vi "StartDataCollection.vi"   [LabVIEW 2011]
uses:
  GlobalVariables.vi
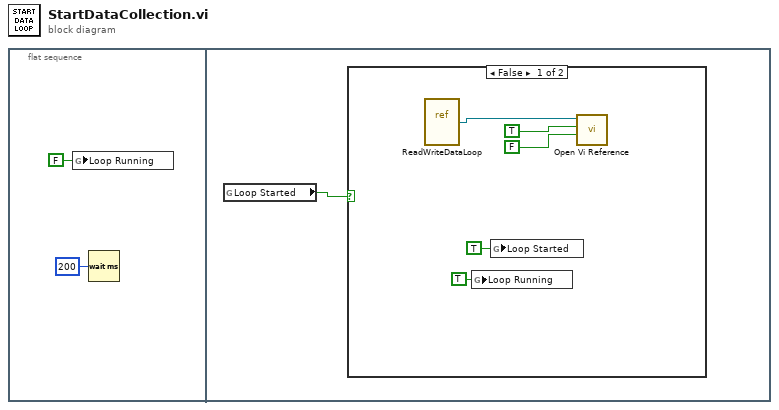
[diagram p0: block diagram]
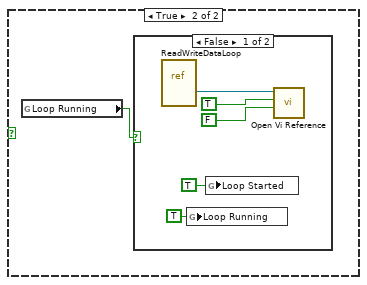
[diagram p2: hidden frame]
diagram:
  n1 = flat-sequence {
    frame #0 {
      n2 = global write "GlobalVariables.vi" "Loop Running"(FALSE ("Loop Running")) -> ()
      n3 = Wait (ms)(milliseconds to wait=u32 200) -> ()  [unwired: 1 out]
    }
    frame #1 {
      n4 = global read "GlobalVariables.vi" "Loop Started"() -> (w3:bool)
      n5 = case shown="False" w3 {
        frame False {
          n6 = vi-ref "ReadWriteDataLoop.vi"() -> (w6:refnum<vi>)
          n7 = global write "GlobalVariables.vi" "Loop Running"(TRUE ("Loop Started")) -> ()
          n8 = global write "GlobalVariables.vi" "Loop Started"(TRUE ("Loop Started")) -> ()
          n9 = call "Open Vi Reference.vi"("Show"=FALSE, "RunVi"=TRUE, "reference"=w6) -> ()  [unwired: 1 in, 2 out]
        }
        frame True {
          n10 = global read "GlobalVariables.vi" "Loop Running"() -> (w9:bool)
          n11 = case shown="False" w9 {
            frame False {
              n12 = vi-ref "ReadWriteDataLoop.vi"() -> (w12:refnum<vi>)
              n13 = global write "GlobalVariables.vi" "Loop Running"(TRUE ("Loop Started")) -> ()
              n14 = global write "GlobalVariables.vi" "Loop Started"(TRUE ("Loop Started")) -> ()
              n15 = call "Open Vi Reference.vi"("Show"=FALSE, "RunVi"=TRUE, "reference"=w12) -> ()  [unwired: 1 in, 2 out]
            }
            frame True {
            }
          }
        }
      }
    }
  }
